vi "Build Assert VI.vi"(8 "error in (no error)":errorcluster, 10 "Type":T5=enum."Double Float", 11 "VI Refnum":refnum<vi>) -> (0 "error out":errorcluster, 2 "Add Object":bool, 3 "Assert VI Path":path, 5 "Assert Add Configuration":T1)   [LabVIEW 2018]
doc: "Dialog box which shows up and dynamically reconfigures during the process of creating a new assert"
uses:
  Numeric Operations.ctl
  <vilib>/Utility/Data Type/Type Definitions/Data Type.ctl
  String Operations.ctl
  Assert Add Configuration.ctl
  FP UI References.ctl
  Assert Scripting Configuration.ctl
  Test Classes/Test.lvclass
  Test Classes/Floating Point/Floating Point.lvclass
  C:/Users/UKHornP/Documents/Work/Projects/Assert_API/Plugins/Utility/Test Classes/Test.lvclass
  Test Classes/String/String.lvclass
  Test Classes/Integer/Integer.lvclass
  Test Classes/Boolean/Boolean.lvclass
  Save VI Ref Source.ctl
  Test Classes/Test.lvclass/Test.ctl
  <vilib>/event_ctls.llb/eventvkey.ctl
  Test Classes/Floating Point/Floating Point.lvclass/Floating Point.ctl
  9e82a159-5312-41f2-9a51-717d948ffea4.vi
  <vilib>/JDP Science/JSONtext/Find Item.vi
  9e82a159-5312-41f2-9a51-717d948ffea4.vi/5f7c14fc-934d-4ccf-ad63-af3d4d4c1745.vi
  <vilib>/JDP Science/JSONtext/String Subset.vi
  Wizard Config/Wizard Strings.vi
  Wizard Config/Create Default Wizard Configuration.vi
  <vilib>/JDP Science/JSONtext/Parsing/Parse Full Path or Item Name.vi
  <vilib>/JDP Science/JSONtext/Offset/Find Item Locations by Path.vi
  <vilib>/JDP Science/JSONtext/JSON text to Variant.vi
  Test Classes/Test Class String IDs.vi
  <vilib>/Utility/Data Type/NI_Data Type.lvlib
panel:
  in  "Settings":bool
  out "<JSON>":string
  in  "Invert Result?":bool
  in  "Include Evaluation String Comment":bool=TRUE
  in  "Digits of Precision":u8=6
  in  "I64 Comparison Value 2":i64 caption="Comparison Value"
  in  "I16 Comparison Value 2":i16 caption="Comparison Value"
  in  "I8 Comparison Value 2":i8 caption="Comparison Value"
  in  "U64 Comparison Value 2":u64 caption="Comparison Value"
  in  "U32 Comparison Value 2":u32 caption="Comparison Value"
  in  "U16 Comparison Value 2":u16 caption="Comparison Value"
  in  "U8 Comparison Value 2":u8 caption="Comparison Value"
  in  "U64 Comparison Value 1":u64
  in  "U32 Comparison Value 1":u32
  in  "U16 Comparison Value 1":u16
  in  "U8 Comparison Value 1":u8
  in  "I64 Comparison Value 1":i64
  in  "I16 Comparison Value 1":i16
  in  "I8 Comparison Value 1":i8
  in  "EXT Comparison Value 2":ext caption="Comparison Value"
  in  "EXT Comparison Value 1":ext
  in  "SGL Comparison Value 2":sgl caption="Comparison Value"
  in  "SGL Comparison Value 1":sgl
  in  "Boolean Comparison Value":bool caption="Comparison Value"
  in  "String Operations":T2 caption="Operation"
  in  "Operation":T3="EQ"
  in  "Default Failure Action":T4(ring)
  in  "Description":string
  in  "String Comparison Value":string caption="Comparison Value"
  in  "I32 Comparison Value 1":i32
  in  "DBL Comparison Value 1":dbl
  in  "Comment":string
  in  "Assert Name":string
  in  "Create":bool
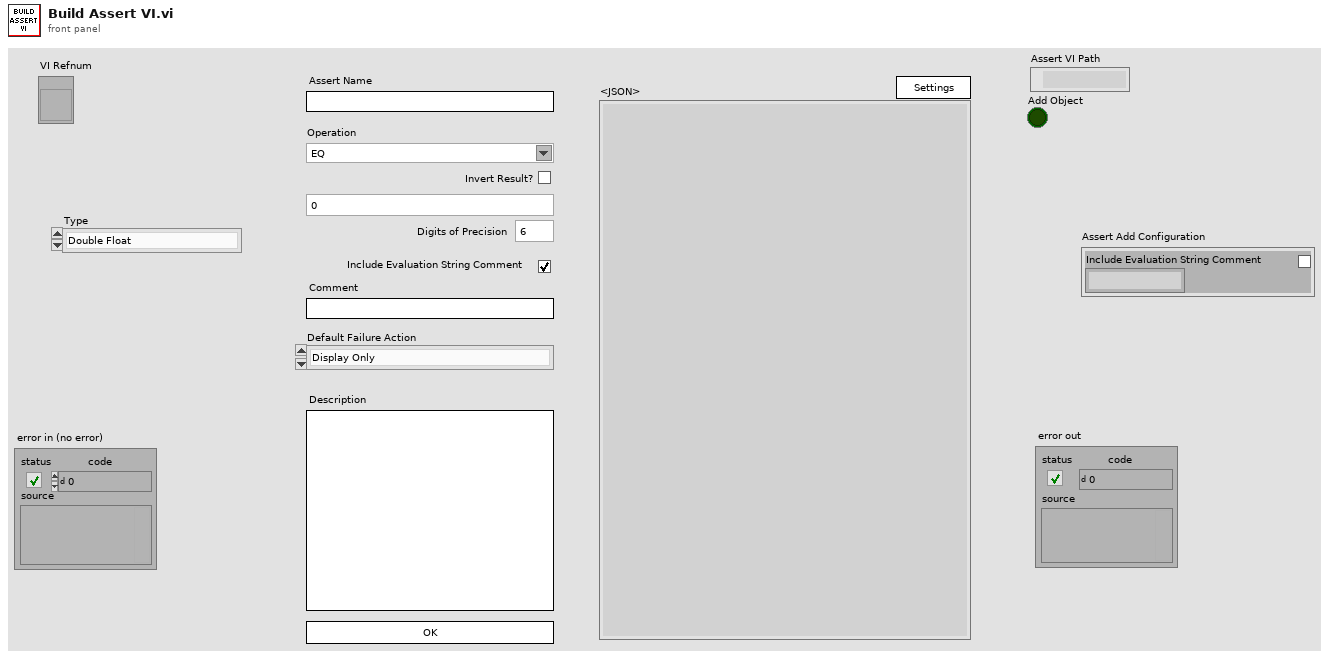
[diagram p1: front panel]
types:
  T1 = typedef "Assert Add Configuration.ctl" = cluster{"Include Evaluation String Comment":bool, "Eval String":string}
  T2 = typedef "String Operations.ctl" = string
  T3 = typedef "Numeric Operations.ctl" = string
  T4 = enum16{"Display Only", "Log To File", "Pause Execution", "Abort Execution"}
  T5 = typedef "NI_Data Type.lvlib/Data Type.ctl" = enum8{"Invalid Type", "Void", "I8", "I16", "I32", "I64", "U8", "U16", "U32", "U64", "Single Float", "Double Float", "Extended Float", "Single Complex", "Double Complex", "Extended Complex", "Enum U8", "Enum U16", "Enum U32", "Enum U64", "Single Float With Unit", "Double Float With Unit", "Extended Float With Unit", "Single Complex with Unit", "Double Complex with Unit", "Extended Complex with Unit", "Boolean", "String", "Path", "Picture", "Tag", "Array", "Cluster", "Variant", "LV Variant", "Waveform", "Timestamp", "Digital Waveform", "Digital Data", "ExpressData", "Refnum", "External Data", "VI", "Poly VI", "LabVIEW Class Instance", "Fixed Point"}
  T6 = typedef "FP UI References.ctl" = cluster{"String Comparison Value":refnum<vi>, "DBL Comparison Value 1":refnum<vi>, "I32 Comparison Value 1":refnum<vi>, "String Operation":refnum<vi>, "Numeric Operation":refnum<vi>, "Boolean Comparison Value":refnum<vi>, "I8 Comparison Value 1":refnum<vi>, "I16 Comparison Value 1":refnum<vi>, "I64 Comparison Value 1":refnum<vi>, "U16 Comparison Value 1":refnum<vi>, "U8 Comparison Value 1":refnum<vi>, "U32 Comparison Value 1":refnum<vi>, "U64 Comparison Value 1":refnum<vi>, "SGL Comparison Value 1":refnum<vi>, "EXT Comparison Value 1":refnum<vi>, "Float Digits of Precision":refnum<vi>}
  T7 = typedef "Assert Scripting Configuration.ctl" = cluster{"Assert Name":string, "Comment":string, "Numeric Operation":string, "Type":T5, "String Operation":string, "DBL Comparison Value 1":dbl, "DBL Comparison Value 2":dbl, "I32 Comparison Value 1":i32, "I32 Comparison Value 2":i32, "String Comparison Value":string, "Description":string, "Default Failure Action":enum16{"Display Only", "Log To File", "Pause Execution", "Abort Execution"}, "Boolean Comparison Value":bool, "I8 Comparison Value 1":i8, "I8 Comparison Value 2":i8, "I16 Comparison Value 1":i16, "I16 Comparison Value 2":i16, "I64 Comparison Value 1":i64, "I64 Comparison Value 2":i64, "U8 Comparison Value 1":u8, "U8 Comparison Value 2":u8, "U16 Comparison Value 1":u16, "U16 Comparison Value 2":u16, "U32 Comparison Value 1":u32, "U32 Comparison Value 2":u32, "U64 Comparison Value 1":u64, "U64 Comparison Value 2":u64, "EXT Comparison Value 1":ext, "EXT Comparison Value 2":ext, "SGL Comparison Value 1":sgl, "SGL Comparison Value 2":sgl, "Float Digits of Precision":u8, "Test Specific Config":refnum<class "Test.lvclass">}
  T8 = typedef "Save VI Ref Source.ctl" = enum16{"File Path", "VI Reference"}
  T9 = typedef "eventvkey.ctl" = enum16{"ASCII", "Enter", "Return", "Shift", "Ctrl", "Alt", "Cmd", "Opt", "Caps", "NumLock", "Clear", "Break", "Up", "Down", "Left", "Right", "Insert", "Delete", "Home", "End", "PageUp", "PageDown", "Escape", "Help", "Pause", "ScrollLock", "F1", "F2", "F3", "F4", "F5", "F6", "F7", "F8", "F9", "F10", "F11", "F12", "F13", "F14", "F15", "F16", "F17", "F18", "F19", "F20", "F21", "F22", "F23", "F24", "Play", "VolumeUp", "VolumeDown", "Mute", "Two Byte Char"}
  T10 = cluster{"Comparison Value 1":string, "Comparison Value 2":string, "Invert Result":string, "Assert VI Name":string, "Data Type":string, "Builder User Name":string, "Build Timestamp":string, "Failure Action":string, "Comment":string, "Assert Name":string, "Description":string, "Evaluation String":string}
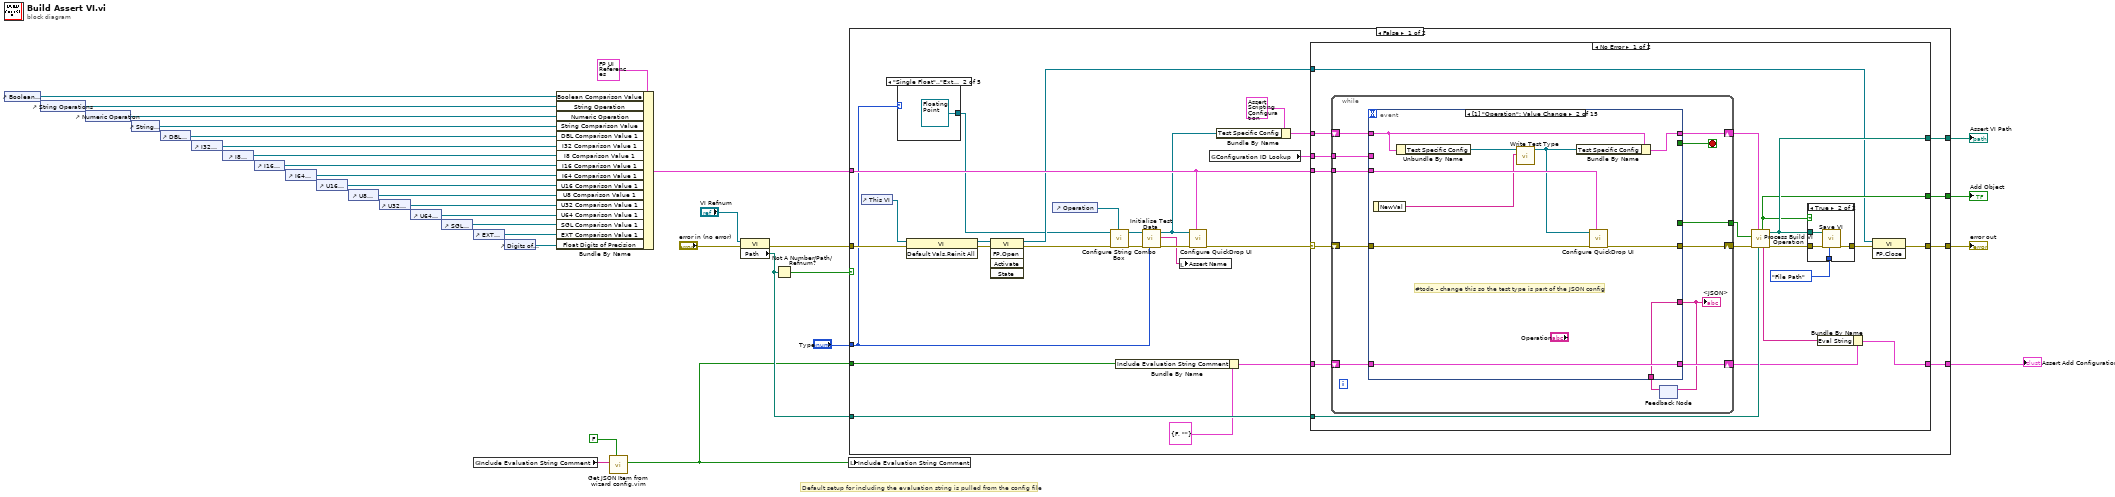
[diagram p0: block diagram]
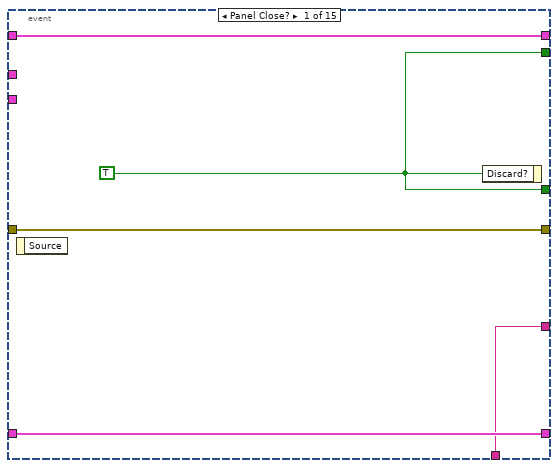
[diagram p3: hidden frame]
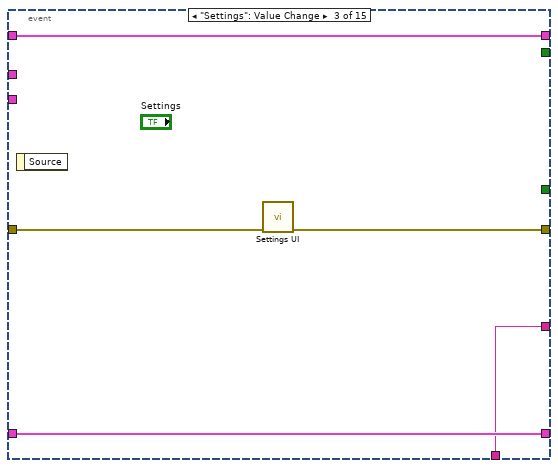
[diagram p4: hidden frame]
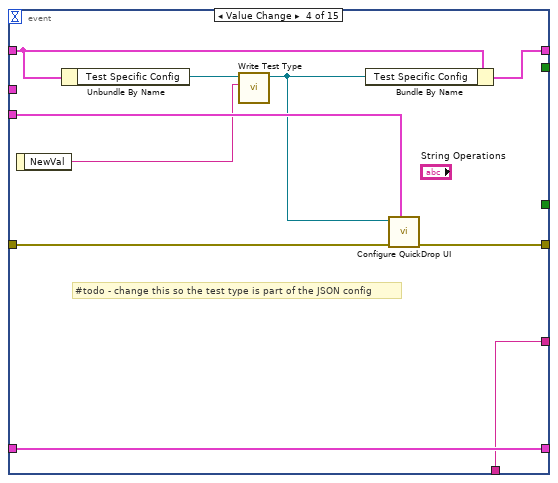
[diagram p5: hidden frame]
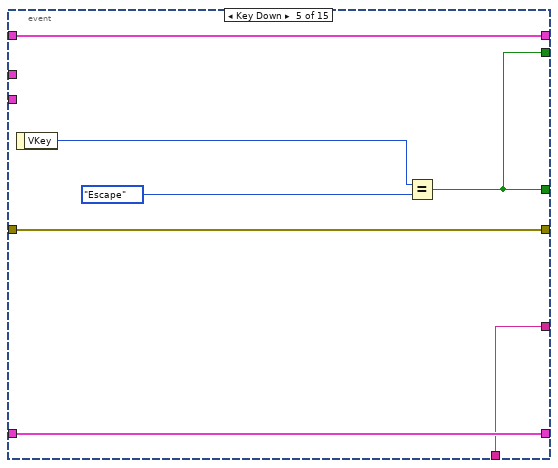
[diagram p6: hidden frame]
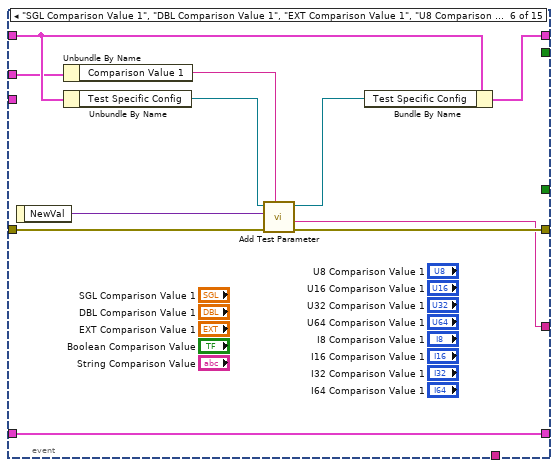
[diagram p7: hidden frame]
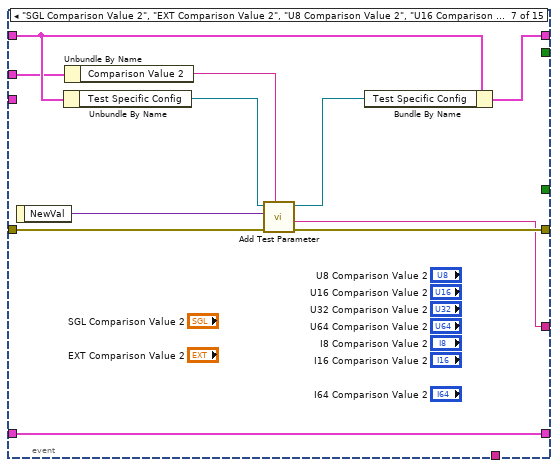
[diagram p8: hidden frame]
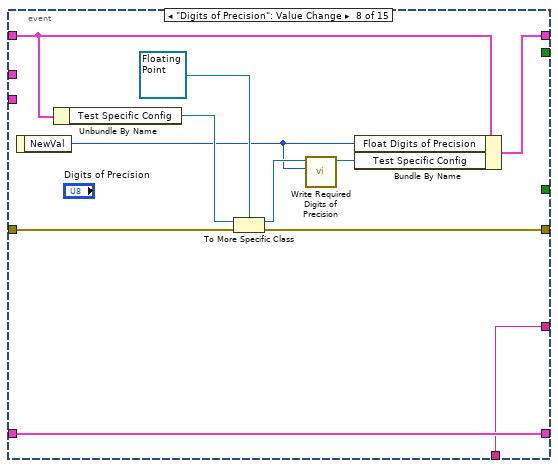
[diagram p9: hidden frame]
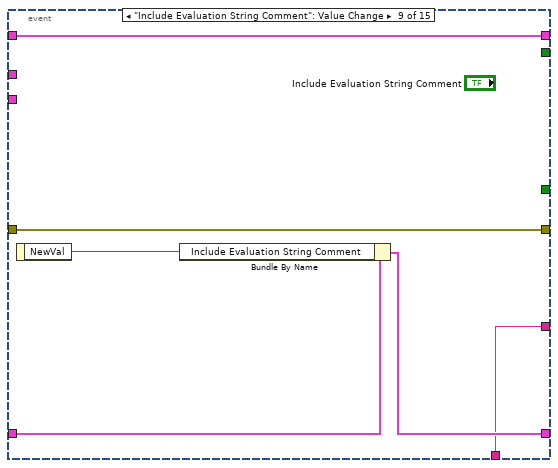
[diagram p10: hidden frame]
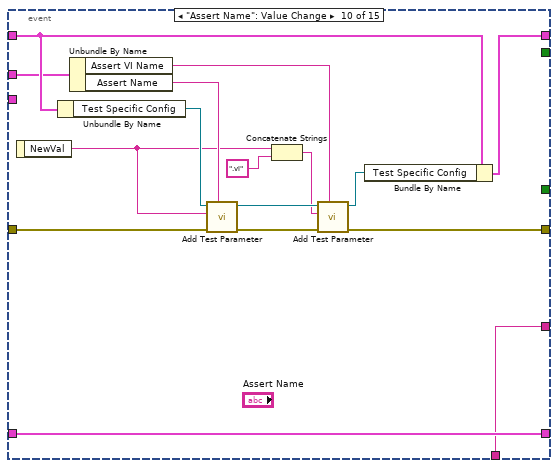
[diagram p11: hidden frame]
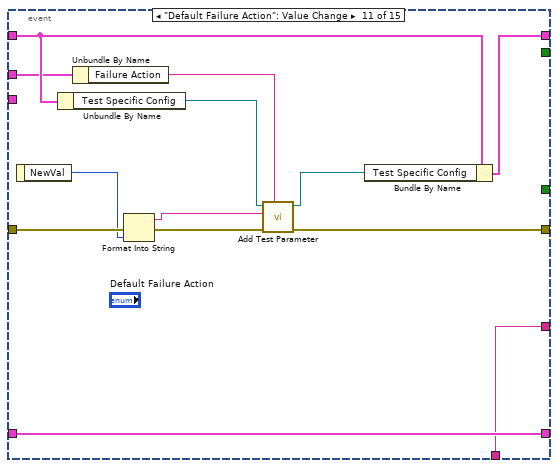
[diagram p12: hidden frame]
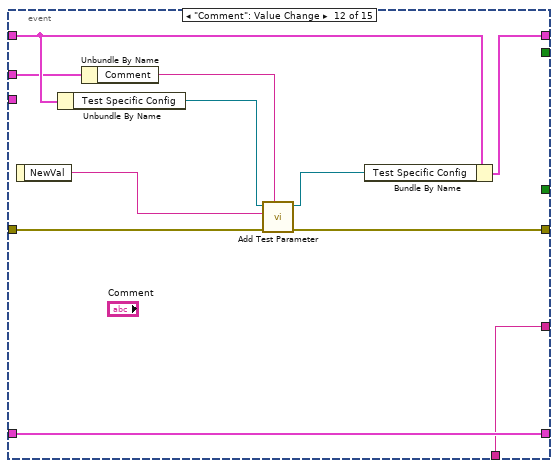
[diagram p13: hidden frame]
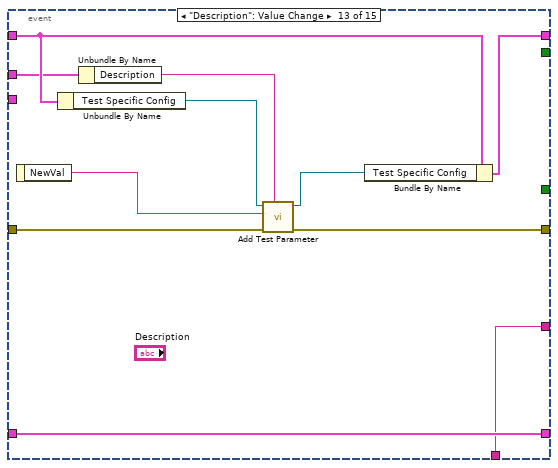
[diagram p14: hidden frame]
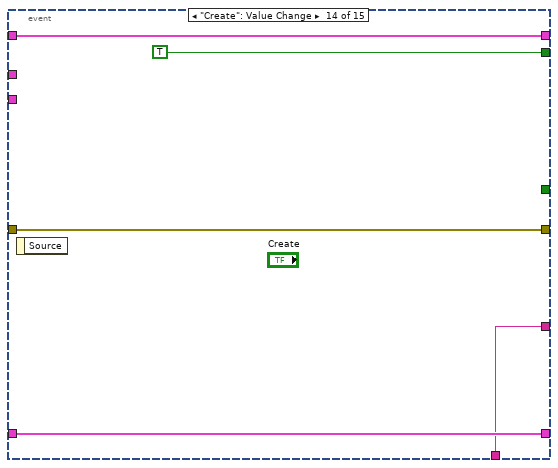
[diagram p15: hidden frame]
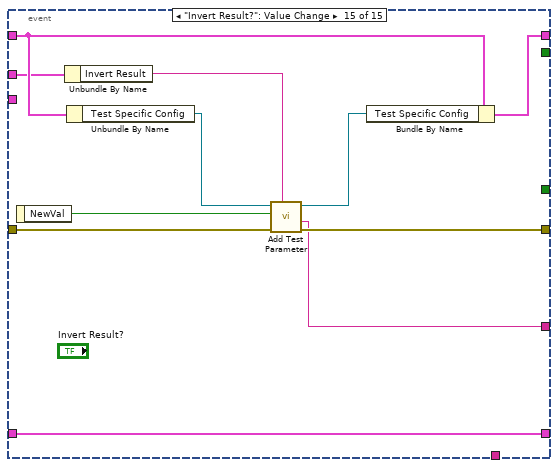
[diagram p16: hidden frame]
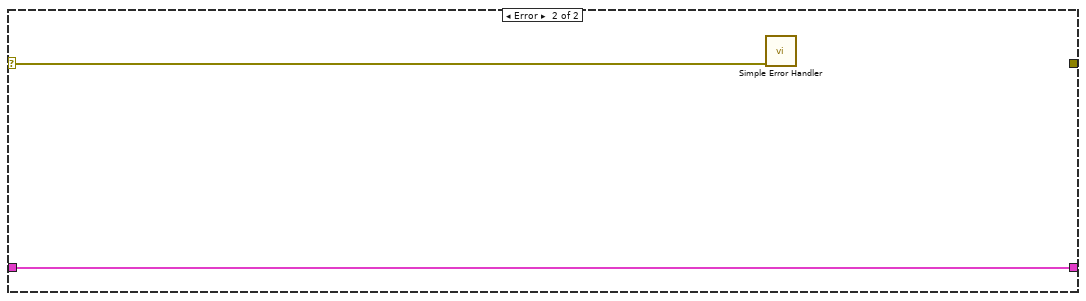
[diagram p17: hidden frame]
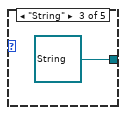
[diagram p19: hidden frame]
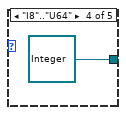
[diagram p20: hidden frame]
diagram:
  # "Default setup for including the evaluation string is pulled from the config file"
  n1 = control-ref of="Boolean Comparison Value"() -> (w25:refnum<vi>)
  n2 = control-ref of="String Operations"() -> (w24:refnum<vi>)
  n3 = control-ref of="Numeric Operation"() -> (w23:refnum<vi>)
  n4 = control-ref of="String Comparison Value"() -> (w21:refnum<vi>)
  n5 = control-ref of="DBL Comparison Value 1"() -> (w20:refnum<vi>)
  n6 = control-ref of="I32 Comparison Value 1"() -> (w19:refnum<vi>)
  n7 = control-ref of="I8 Comparison Value 1"() -> (w17:refnum<vi>)
  n8 = control-ref of="I16 Comparison Value 1"() -> (w16:refnum<vi>)
  n9 = control-ref of="I64 Comparison Value 1"() -> (w15:refnum<vi>)
  n10 = control-ref of="U16 Comparison Value 1"() -> (w13:refnum<vi>)
  n11 = control-ref of="U8 Comparison Value 1"() -> (w14:refnum<vi>)
  n12 = control-ref of="U32 Comparison Value 1"() -> (w12:refnum<vi>)
  n13 = control-ref of="U64 Comparison Value 1"() -> (w11:refnum<vi>)
  n14 = control-ref of="SGL Comparison Value 1"() -> (w10:refnum<vi>)
  n15 = control-ref of="EXT Comparison Value 1"() -> (w9:refnum<vi>)
  n16 = global read "Wizard Strings.vi" "Include Evaluation String Comment"() -> (w4:string)
  n17 = control-ref of="Digits of Precision"() -> (w8:refnum<vi>)
  n18 = Bundle By Name(cluster=T6 {"String Comparison Value"=refnum, "DBL Comparison Value 1"=refnum, "I32 Comparison Value 1"=refnum, "String Operation"=refnum, "Numeric Operation"=refnum, "Boolean Comparison Value"=refnum, "I8 Comparison Value 1"=refnum, "I16 Comparison Value 1"=refnum, "I64 Comparison Value 1"=refnum, "U16 Comparison Value 1"=refnum, "U8 Comparison Value 1"=refnum, "U32 Comparison Value 1"=refnum, "U64 Comparison Value 1"=refnum, "SGL Comparison Value 1"=refnum, "EXT Comparison Value 1"=refnum, "Float Digits of Precision"=refnum}, "Boolean Comparison Value"=w25, "String Operation"=w24, "Numeric Operation"=w23, "String Comparison Value"=w21, "DBL Comparison Value 1"=w20, "I32 Comparison Value 1"=w19, "I8 Comparison Value 1"=w17, "I16 Comparison Value 1"=w16, "I64 Comparison Value 1"=w15, "U16 Comparison Value 1"=w13, "U8 Comparison Value 1"=w14, "U32 Comparison Value 1"=w12, "U64 Comparison Value 1"=w11, "SGL Comparison Value 1"=w10, "EXT Comparison Value 1"=w9, "Float Digits of Precision"=w8) -> (w18:T6)
  n19 = call "Get JSON Item from wizard config.vim"("Data Type"=FALSE, "$Path or Item Name"=w4) -> ("<JSON>"=w2:bool)  [unwired: 7 in, 2 out]
  n20 = property class="VI"(reference="VI Refnum", error in="error in (no error)") -> (error out=w6:errorcluster, "Path"=w30:path)  [unwired: 1 out]
  n21 = Not A Number/Path/Refnum?(number/path/refnum=w30) -> (NaN/Path/Refnum?=w1:bool)
  n22 = local write "Include Evaluation String Comment"(w2) -> ()
  n23 = case shown="False" w1 {
    tunnel: w30 -> [w58 _]
    tunnel: w6 -> [w57 w245]
    tunnel: [w38 w245] -> w28
    tunnel: [w54 _] -> w27
    tunnel: [w53 _] -> w26
    tunnel: w18 -> [w49 _]
    tunnel: w2 -> [w44 _]
    tunnel: [w47 _] -> w7
    tunnel: "Type" -> [w39 _]
    frame False {
      n24 = control-ref of="This VI"() -> (w48:refnum<vi>)
      n25 = case shown="\"Single Float\"..\"Extended Float\"" w39 {
        tunnel: [_ refnum<class "Floating Point.lvclass"> refnum ("Floating Point.lvclass") refnum<class "String.lvclass"> refnum ("String.lvclass") refnum<class "Integer.lvclass"> refnum ("Integer.lvclass") refnum<class "Boolean.lvclass"> refnum ("Boolean.lvclass")] -> w34
        frame "Invalid Type", Default {
        }
        frame "Single Float".."Extended Float" {
        }
        frame "String" {
        }
        frame "I8".."U64" {
        }
        frame "Boolean" {
        }
      }
      n26 = invoke class="VI" method="Default Vals.Reinit All"(reference=w48, error in=w57) -> (reference out=w55:refnum<vi>, error out=w56:errorcluster)  [unwired: 1 in, 1 out]
      n27 = invoke class="VI" method="FP.Open"(reference=w55, error in=w56) -> (reference out=w37:refnum<vi>, error out=w43:errorcluster)  [unwired: 3 in, 3 out]
      n28 = control-ref of="Operation"() -> (w32:refnum<vi>)
      n29 = call "Configure String Combo Box.vi"("Operation Ctrl Ref"=w32, "error in (no error)"=w43, "Test in"=w34) -> ("error out"=w35:errorcluster, "Test out"=w33:refnum<class "Test.lvclass">)  [unwired: 7 in]
      n30 = Bundle By Name(cluster=T1 {"Include Evaluation String Comment"=FALSE, "Eval String"=""} ("Assert Add Configuration"), "Include Evaluation String Comment"=w44) -> (w45:T1)
      n31 = call "Initialise Test Data.vi"("Data Type"=w39, "error in (no error)"=w35, "Test in"=w33) -> ("error out"=w41:errorcluster, "Assert Name"=w36:string, "Test out"=w40:refnum<class "Test.lvclass">)  [unwired: 6 in]
      n32 = local write "Assert Name"(w36) -> ()
      n33 = call "Configure QuickDrop UI.vi"("FP UI References"=w49, "error in (no error)"=w41, "Test in"=w40) -> ("error out"=w52:errorcluster)  [unwired: 8 in]
      n34 = global read "Test Class String IDs.vi" "Configuration ID Lookup"() -> (w42:T10)
      n35 = Bundle By Name(cluster=T7 {"Assert Name"="", "Comment"="", "Numeric Operation"="", "Type"=enum."Double Float", "String Operation"="", "DBL Comparison Value 1"=0.0, "DBL Comparison Value 2"=0.0, "I32 Comparison Value 1"=0, "I32 Comparison Value 2"=0, "String Comparison Value"="", "Description"="", "Default Failure Action"=enum."Display Only", "Boolean Comparison Value"=FALSE, "I8 Comparison Value 1"=0, "I8 Comparison Value 2"=0, "I16 Comparison Value 1"=0, "I16 Comparison Value 2"=0, "I64 Comparison Value 1"=0, "I64 Comparison Value 2"=0, "U8 Comparison Value 1"=0, "U8 Comparison Value 2"=0, "U16 Comparison Value 1"=0, "U16 Comparison Value 2"=0, "U32 Comparison Value 1"=0, "U32 Comparison Value 2"=0, "U64 Comparison Value 1"=0, "U64 Comparison Value 2"=0, "EXT Comparison Value 1"=0.0, "EXT Comparison Value 2"=0.0, "SGL Comparison Value 1"=0.0, "SGL Comparison Value 2"=0.0, "Float Digits of Precision"=0, "Test Specific Config"=refnum}, "Test Specific Config"=w40) -> (w50:T7)
      n36 = case shown="No Error" w52 {
        selector: w52 -> [w76 w239]
        tunnel: w58 -> [w73 _]
        tunnel: [w60 _] -> w38
        tunnel: [w68 _] -> w54
        tunnel: [w67 _] -> w53
        tunnel: w50 -> [w75 _]
        tunnel: w49 -> [w72 _]
        tunnel: [w64 w238] -> w47
        tunnel: w45 -> [w66 w238]
        tunnel: w42 -> [w61 _]
        tunnel: w37 -> [w59 _]
        frame No Error {
          n37 = while {
            tunnel: [w94] -> w74
            shift-right: [w93] -> w70
            shift-left: w76 -> [w92]
            shift-right: [w89] -> w71
            shift-left: w75 -> [w90]
            tunnel: w72 -> [w88]
            shift-right: [w87] -> w65
            shift-left: w66 -> [w86]
            tunnel: w61 -> [w83]
            stop <- w91 stop-if-true
            n38 = feedback #1() -> (w85:string)  [unwired: 1 in]
            n39 = event shown="[1] \"Operation\": Value Change" {
              selector: _ -> [_ _ _ _ _ _ _ _ _ _ _ _ _ _ _]
              dyn-events: _ -> [_ _ _ _ _ _ _ _ _ _ _ _ _ _ _]
              timeout: _ -> [_ _ _ _ _ _ _ _ _ _ _ _ _ _ _]
              tunnel: [w98 _ _ _ w128 _ _ _ _ _ _ _ _ _ _] -> w94
              tunnel: w92 -> [w99 w109 w111 w124 w127 w142 w153 w157 w169 w185 w198 w209 w220 w226 w236]
              tunnel: [w99 w107 w110 w122 w127 w138 w149 w156 w169 w177 w195 w206 w217 w226 w234] -> w93
              tunnel: [w98 _ _ _ w128 _ _ _ _ _ _ _ _ TRUE _] -> w91
              tunnel: w90 -> [w97 w104 w114 w119 w131 w139 w150 w162 w170 w181 w194 w205 w216 w224 w233]
              tunnel: [w97 w108 w114 w123 w131 w141 w152 w164 w170 w186 w199 w210 w221 w224 w235] -> w89
              tunnel: w88 -> [_ w106 _ w121 _ _ _ _ _ _ _ _ _ _ _]
              tunnel: [w96 w105 w113 w120 w126 w140 w151 w163 w168 w184 w197 w208 w219 w223 w237] -> w87
              tunnel: w86 -> [w96 w105 w113 w120 w126 w140 w151 w163 w167 w184 w197 w208 w219 w223 w237]
              tunnel: [w95 w100 w112 w115 w125 w134 w145 w154 w165 w183 w196 w207 w218 w222 w229] -> w84
              tunnel: w85 -> [w95 w100 w112 w115 w125 _ _ w154 w165 w183 w196 w207 w218 w222 _]
              tunnel: w83 -> [_ _ _ _ _ w133 w144 _ _ w180 w193 w204 w215 _ w228]
              event Panel Close? {
                w98 = TRUE ("Discard?")
                n40 = event-data() -> ()  [unwired: 1 in, 1 out]
                n41 = event-data("Discard?"=w98) -> ()  [unwired: 1 in, 1 out]
              }
              event Value Change {
                # "#todo - change this so the test type is part of the JSON config"
                n42 = event-data() -> ("NewVal"=w102:T3)  [unwired: 1 in]
                n43 = Unbundle By Name(w104) -> ("Test Specific Config"=w103:refnum<class "Test.lvclass">)
                n44 = call "Write Test Type.vi"("Test Type"=w102, "Test in"=w103) -> ("Test out"=w101:refnum<class "Test.lvclass">)  [unwired: 9 in]
                n45 = Bundle By Name(cluster=w104, "Test Specific Config"=w101) -> (w108:T7)
                n46 = call "Configure QuickDrop UI.vi"("FP UI References"=w106, "error in (no error)"=w109, "Test in"=w101) -> ("error out"=w107:errorcluster)  [unwired: 8 in]
              }
              event "Settings": Value Change {
                n47 = event-data() -> ()  [unwired: 1 in, 1 out]
                n48 = call "Settings UI.vi"("error in (no error)"=w111) -> ("error out"=w110:errorcluster)  [unwired: 10 in]
              }
              event Value Change {
                # "#todo - change this so the test type is part of the JSON config"
                n49 = event-data() -> ("NewVal"=w117:T2)  [unwired: 1 in]
                n50 = Unbundle By Name(w119) -> ("Test Specific Config"=w118:refnum<class "Test.lvclass">)
                n51 = call "Write Test Type.vi"("Test Type"=w117, "Test in"=w118) -> ("Test out"=w116:refnum<class "Test.lvclass">)  [unwired: 9 in]
                n52 = Bundle By Name(cluster=w119, "Test Specific Config"=w116) -> (w123:T7)
                n53 = call "Configure QuickDrop UI.vi"("FP UI References"=w121, "error in (no error)"=w124, "Test in"=w116) -> ("error out"=w122:errorcluster)  [unwired: 8 in]
              }
              event Key Down {
                n54 = event-data() -> ("VKey"=w130:T9)  [unwired: 1 in]
                n55 = Equal?(x=w130, y=eventvkey."Escape") -> (x = y?=w128:bool)
              }
              event "SGL Comparison Value 1", "DBL Comparison Value 1", "EXT Comparison Value 1", "U8 Comparison Value 1", "U16 Comparison Value 1", "U32 Comparison Value 1", "U64 Comparison Value 1", "I8 Comparison Value 1", "I16 Comparison Value 1", "I32 Comparison Value 1", "I64 Comparison Value 1", "Boolean Comparison Value", "String Comparison Value": Value Change {
                n56 = event-data() -> ("NewVal"=w135:variant)  [unwired: 1 in]
                n57 = Unbundle By Name(w133) -> ("Comparison Value 1"=w132:string)
                n58 = Unbundle By Name(w139) -> ("Test Specific Config"=w136:refnum<class "Test.lvclass">)
                n59 = call-dynamic "Add Test Parameter.vi"("Data Value ID"=w132, "error in (no error)"=w142, "Data Value"=w135, "Test in"=w136) -> ("error out"=w138:errorcluster, "<JSON>"=w134:string, "Test out"=w137:refnum<class "Test.lvclass">)  [unwired: 5 in]
                n60 = Bundle By Name(cluster=w139, "Test Specific Config"=w137) -> (w141:T7)
              }
              event "SGL Comparison Value 2", "EXT Comparison Value 2", "U8 Comparison Value 2", "U16 Comparison Value 2", "U32 Comparison Value 2", "U64 Comparison Value 2", "I8 Comparison Value 2", "I16 Comparison Value 2", "I64 Comparison Value 2": Value Change {
                n61 = event-data() -> ("NewVal"=w146:variant)  [unwired: 1 in]
                n62 = Unbundle By Name(w150) -> ("Test Specific Config"=w147:refnum<class "Test.lvclass">)
                n63 = Unbundle By Name(w144) -> ("Comparison Value 2"=w143:string)
                n64 = call-dynamic "Add Test Parameter.vi"("Data Value ID"=w143, "error in (no error)"=w153, "Data Value"=w146, "Test in"=w147) -> ("error out"=w149:errorcluster, "<JSON>"=w145:string, "Test out"=w148:refnum<class "Test.lvclass">)  [unwired: 5 in]
                n65 = Bundle By Name(cluster=w150, "Test Specific Config"=w148) -> (w152:T7)
              }
              event "Digits of Precision": Value Change {
                n66 = event-data() -> ("NewVal"=w158:u8)  [unwired: 1 in]
                n67 = Unbundle By Name(w162) -> ("Test Specific Config"=w161:refnum<class "Test.lvclass">)
                n68 = To More Specific Class(target class=refnum<class "Floating Point.lvclass"> refnum ("Floating Point.lvclass"), reference=w161, error in=w157) -> (specific class reference=w159:refnum<class "Floating Point.lvclass">, error out=w156:errorcluster)
                n69 = call "Write Required Digits of Precision.vi"("Required Digits of Precision"=w158, "Floating Point in"=w159) -> ("Floating Point out"=w155:refnum<class "Floating Point.lvclass">)  [unwired: 9 in]
                n70 = Bundle By Name(cluster=w162, "Float Digits of Precision"=w158, "Test Specific Config"=w155) -> (w164:T7)
              }
              event "Include Evaluation String Comment": Value Change {
                n71 = event-data() -> ("NewVal"=w166:bool)  [unwired: 1 in]
                n72 = Bundle By Name(cluster=w167, "Include Evaluation String Comment"=w166) -> (w168:T1)
              }
              event "Assert Name": Value Change {
                n73 = event-data() -> ("NewVal"=w173:string)  [unwired: 1 in]
                n74 = Unbundle By Name(w181) -> ("Test Specific Config"=w178:refnum<class "Test.lvclass">)
                n75 = Unbundle By Name(w180) -> ("Assert VI Name"=w174:string, "Assert Name"=w179:string)
                n76 = call-dynamic "Add Test Parameter.vi"("Data Value ID"=w179, "error in (no error)"=w185, "Data Value"=w173, "Test in"=w178) -> ("error out"=w182:errorcluster, "Test out"=w176:refnum<class "Test.lvclass">)  [unwired: 5 in, 1 out]
                n77 = Concatenate Strings(w173, ".vi" ("string")) -> (w171:string)
                n78 = call-dynamic "Add Test Parameter.vi"("Data Value ID"=w174, "error in (no error)"=w182, "Data Value"=w171, "Test in"=w176) -> ("error out"=w177:errorcluster, "Test out"=w175:refnum<class "Test.lvclass">)  [unwired: 5 in, 1 out]
                n79 = Bundle By Name(cluster=w181, "Test Specific Config"=w175) -> (w186:T7)
              }
              event "Default Failure Action": Value Change {
                n80 = event-data() -> ("NewVal"=w188:T4)  [unwired: 1 in]
                n81 = Unbundle By Name(w194) -> ("Test Specific Config"=w191:refnum<class "Test.lvclass">)
                n82 = Unbundle By Name(w193) -> ("Failure Action"=w192:string)
                n83 = Format Into String(error in=w198, w188) -> (resulting string=w187:string, error out=w189:errorcluster)  [unwired: 2 in]
                n84 = call-dynamic "Add Test Parameter.vi"("Data Value ID"=w192, "error in (no error)"=w189, "Data Value"=w187, "Test in"=w191) -> ("error out"=w195:errorcluster, "Test out"=w190:refnum<class "Test.lvclass">)  [unwired: 5 in, 1 out]
                n85 = Bundle By Name(cluster=w194, "Test Specific Config"=w190) -> (w199:T7)
              }
              event "Comment": Value Change {
                n86 = event-data() -> ("NewVal"=w200:string)  [unwired: 1 in]
                n87 = Unbundle By Name(w205) -> ("Test Specific Config"=w202:refnum<class "Test.lvclass">)
                n88 = Unbundle By Name(w204) -> ("Comment"=w203:string)
                n89 = call-dynamic "Add Test Parameter.vi"("Data Value ID"=w203, "error in (no error)"=w209, "Data Value"=w200, "Test in"=w202) -> ("error out"=w206:errorcluster, "Test out"=w201:refnum<class "Test.lvclass">)  [unwired: 5 in, 1 out]
                n90 = Bundle By Name(cluster=w205, "Test Specific Config"=w201) -> (w210:T7)
              }
              event "Description": Value Change {
                n91 = event-data() -> ("NewVal"=w211:string)  [unwired: 1 in]
                n92 = Unbundle By Name(w216) -> ("Test Specific Config"=w213:refnum<class "Test.lvclass">)
                n93 = Unbundle By Name(w215) -> ("Description"=w214:string)
                n94 = call-dynamic "Add Test Parameter.vi"("Data Value ID"=w214, "error in (no error)"=w220, "Data Value"=w211, "Test in"=w213) -> ("error out"=w217:errorcluster, "Test out"=w212:refnum<class "Test.lvclass">)  [unwired: 5 in, 1 out]
                n95 = Bundle By Name(cluster=w216, "Test Specific Config"=w212) -> (w221:T7)
              }
              event "Create": Value Change {
                n96 = event-data() -> ()  [unwired: 1 in, 1 out]
              }
              event "Invert Result?": Value Change {
                n97 = event-data() -> ("NewVal"=w231:bool)  [unwired: 1 in]
                n98 = Unbundle By Name(w228) -> ("Invert Result"=w227:string)
                n99 = Unbundle By Name(w233) -> ("Test Specific Config"=w232:refnum<class "Test.lvclass">)
                n100 = call-dynamic "Add Test Parameter.vi"("Data Value ID"=w227, "error in (no error)"=w236, "Data Value"=w231, "Test in"=w232) -> ("error out"=w234:errorcluster, "<JSON>"=w229:string, "Test out"=w230:refnum<class "Test.lvclass">)  [unwired: 5 in]
                n101 = Bundle By Name(cluster=w233, "Test Specific Config"=w230) -> (w235:T7)
              }
            }
            "<JSON>" <- w84
            n102 = feedback-in #1(w84) -> ()
          }
          n103 = call "Process Build VI Operation.vi"("Caller VI Path"=w73, "Assert Scripting Configuration"=w71, "error in (no error)"=w70, "Discard?"=w74) -> ("error out"=w77:errorcluster, "Assert VI Path"=w68:path, "Evaluation String"=w63:string, "Valid Configuration"=w67:bool)  [unwired: 4 in]
          n104 = case shown="True" w67 {
            tunnel: w77 -> [w78 w82]
            tunnel: [w78 w81] -> w69
            tunnel: w68 -> [_ w80]
            tunnel: Save_VI_Ref_Source."File Path" ("Reference Source") -> [_ w79]
            frame False {
            }
            frame True {
              n105 = call "Save VI.vi"("Reference Source"=w79, "error in (no error)"=w82, "Assert VI Path"=w80) -> ("error out"=w81:errorcluster)  [unwired: 8 in]
            }
          }
          n106 = Bundle By Name(cluster=w65, "Eval String"=w63) -> (w64:T1)
          n107 = invoke class="VI" method="FP.Close"(reference=w59, error in=w69) -> (error out=w60:errorcluster)  [unwired: 1 in, 2 out]
        }
        frame Error {
          n108 = call <vilib>:"Simple Error Handler.vi"("error in (no error)"=w239) -> ()  [unwired: 4 in, 5 out]
        }
      }
    }
    frame True {
      n109 = One Button Dialog(message="Invalid VI Path - No Assert statements can be created\nSave VI") -> ()  [unwired: 1 in, 1 out]
    }
  }
  "error out" <- w28
  "Assert VI Path" <- w27
  "Add Object" <- w26
  "Assert Add Configuration" <- w7
